vi "Close.vi"(8 "error in (no error)":errorcluster, 11 "SMO.InstrumentDriver in":refnum<class "SMO.InstrumentDriver.lvclass">) -> (0 "error out":errorcluster)   [LabVIEW 2013, in "SMO.InstrumentDriver.lvclass"]
uses:
  SMO.InstrumentDriver.lvclass
  <vilib>/JKI/JKI SMO/SMO/SMO.lvclass
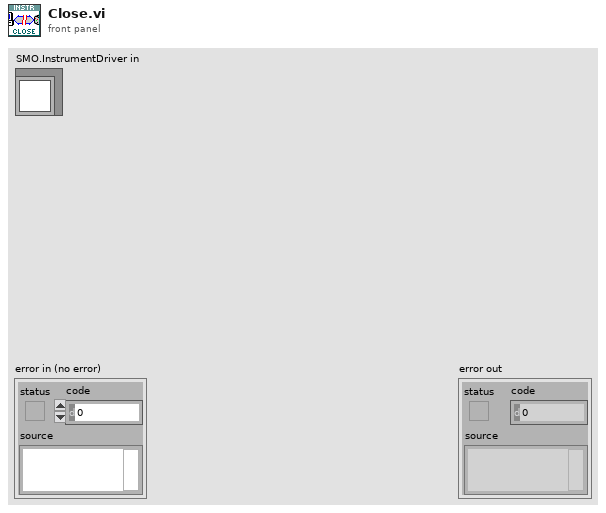
[diagram p1: front panel]
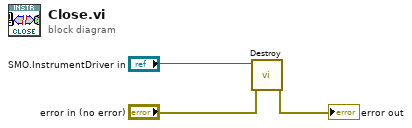
[diagram p0: block diagram]
diagram:
  n1 = call <vilib>:"Destroy.vi"("error in (no error)"="error in (no error)", "SMO"="SMO.InstrumentDriver in") -> ("error out"=→"error out":errorcluster)  [unwired: 9 in]
